vi "Motors.vi"() -> ()   [LabVIEW 2017]
uses:
  <vilib>/Utility/miscctls.llb/LV3DPointTypeDef.ctl
  <vilib>/HaroTek/Haro3D/Utilities/3D objects/controls/Material_info.ctl
  <vilib>/HaroTek/Haro3D/Utilities/3D objects/Box_class/3D_Box.lvclass
  C:/Program Files (x86)/National Instruments/LabVIEW 2017/vi.lib/HaroTek/Haro3D/Utilities/3D objects/3D_Shape_class/3D_Shape.lvclass
  <vilib>/HaroTek/Haro3D/Utilities/3D objects/Cylinder_class/3D_Cylinder.lvclass
  <vilib>/HaroTek/Haro3D/Utilities/3D objects/Sphere_class/3D_Sphere_class/3D_Sphere.lvclass
  <vilib>/HaroTek/Haro3D/Utilities/3D objects/3D_Quad_class/Panel.lvclass
  <vilib>/picture/3D Picture Control/Object/Create Object (name).vi
  <vilib>/picture/3D Picture Control/Object/Add Object (no reference).vi
  <vilib>/HaroTek/Haro3D/Hololens/Hololens_class/Hololens.lvclass
  <vilib>/HaroTek/Haro3D/Hololens/Modules/Hololens Message classes/Text_Message_class/Text_Message.lvclass
  <vilib>/HaroTek/Haro3D/Haro3D.lvlib
  <vilib>/picture/3D Picture Control/NI_3D Picture Control.lvlib
panel:
  in  "TestVar":dbl
  in  "Stop Button":bool
  out "Hololens ON?":bool
  out "3D Picture":refnum<vi>(3d-picture)
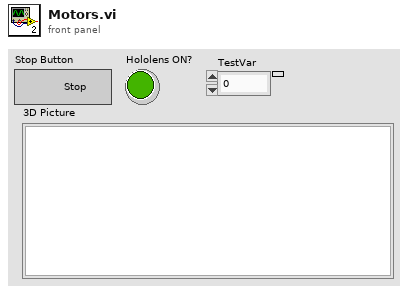
[diagram p1: front panel]
types:
  T1 = typedef "Haro3D.lvlib/Hololens.lvclass/Hololens_event.ctl" = cluster{"Connection":refnum<user-event>, "Data":refnum<user-event>}
  T2 = typedef "LV3DPointTypeDef.ctl" = cluster{"X":sgl, "Y":sgl, "Z":sgl}
  T3 = typedef "Haro3D.lvlib/Material_info.ctl" = cluster{"name":string, "Ka":u32, "Kd":u32, "Ke":u32, "Ks":u32, "map_Ka":string, "map_Kd":string, "map_Ks":string, "Ns":sgl, "Tr":sgl, "UseTexture":bool}
  T4 = typedef "Haro3D.lvlib/Hololens.lvclass/data_event_type.ctl" = enum32{"None", "Mesh", "Text Response", "Manipulation", "Object selected", "Hold", "Receive Anchor", "Sharing", "Secondary connect", "Receive Picture", "Invalid"}
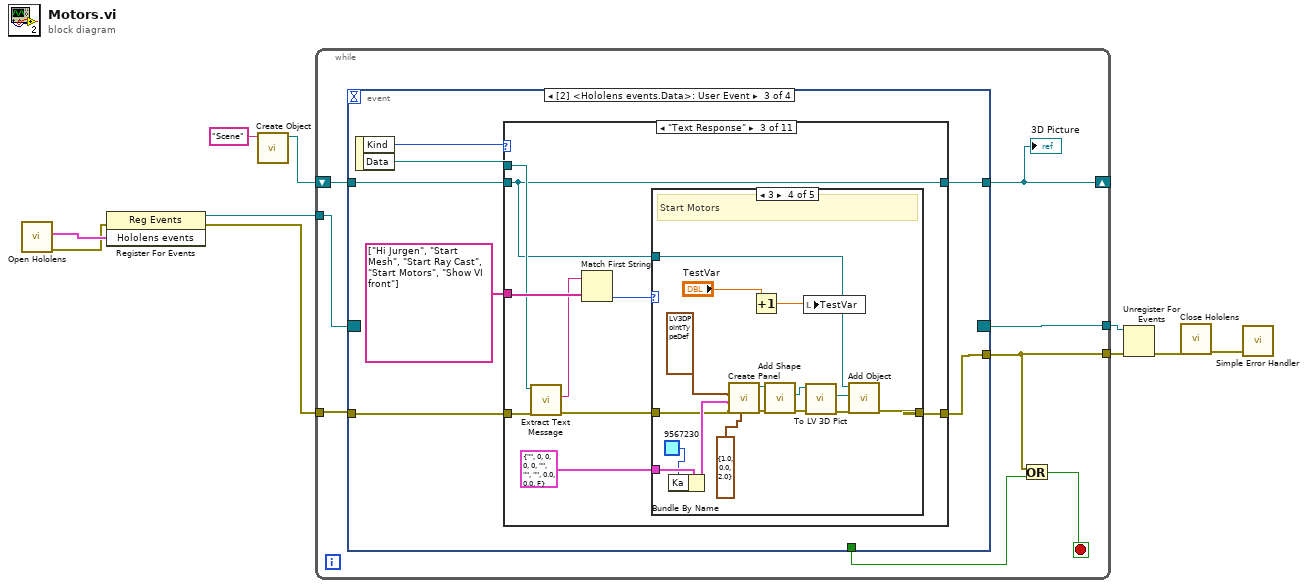
[diagram p0: block diagram]
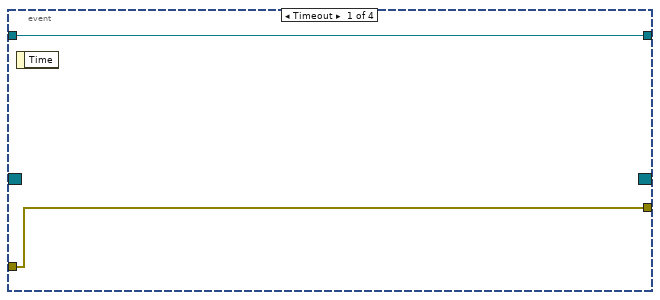
[diagram p2: hidden frame]
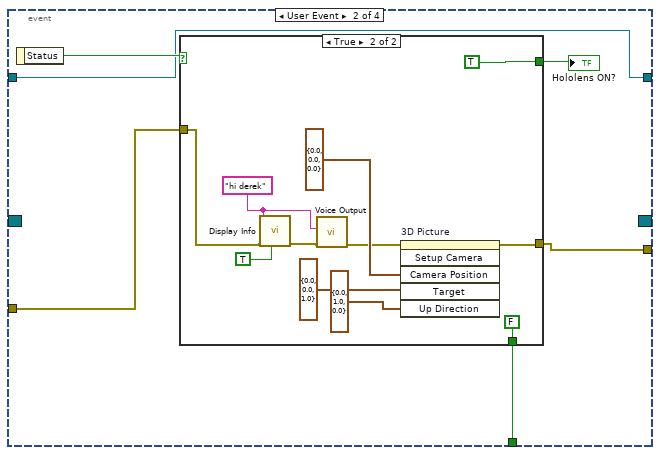
[diagram p3: hidden frame]
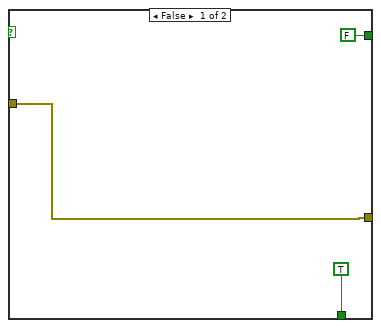
[diagram p4: hidden frame]
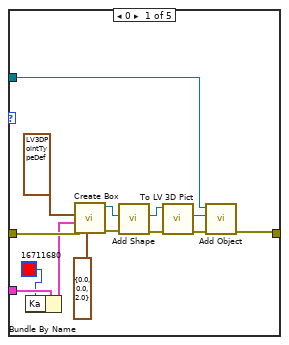
[diagram p7: hidden frame]
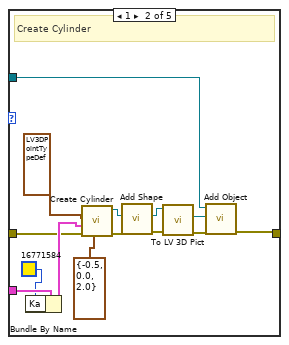
[diagram p8: hidden frame]
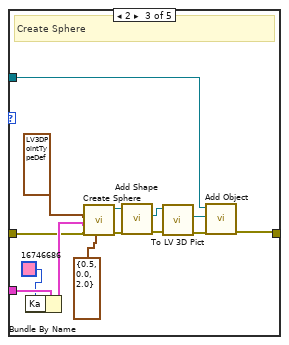
[diagram p9: hidden frame]
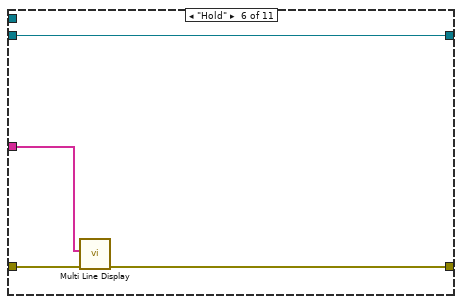
[diagram p13: hidden frame]
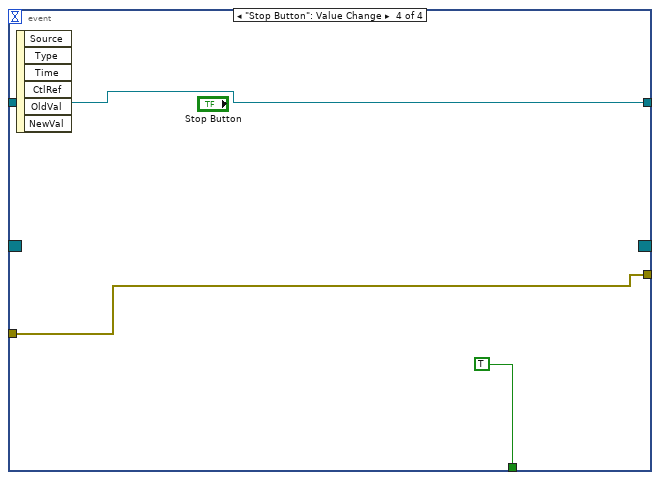
[diagram p19: hidden frame]
diagram:
  n1 = call <vilib>:"Open Hololens.vi"() -> ("error out"=w9:errorcluster, "Hololens events"=w10:T1)  [unwired: 10 in]
  n2 = register-events(error in=w9, w10) -> (reference out=w8:refnum<event-registration>, error out=w7:errorcluster)  [unwired: 1 in]
  n3 = call-poly <vilib>:"Create Object.vi"("Name"="Scene") -> ("Scene:New Object"=w1:refnum<vi>)  [unwired: 9 in, 1 out]
  n4 = while {
    tunnel: w8 -> [w18]
    tunnel: w7 -> [w17]
    tunnel: [w14] -> w6
    tunnel: [w16] -> w4
    shift-right: [w11] -> _
    shift-left: w1 -> [w12]
    stop <- w13 stop-if-true
    n5 = event shown="[2] <Hololens events.Data>: User Event" {
      selector: w18 -> [_ _ _ _]
      dyn-events: [_ _ _ _] -> w16
      timeout: _ -> [_ _ _ _]
      tunnel: w17 -> [w19 w25 w46 w140]
      tunnel: [_ w23 _ TRUE] -> w15
      tunnel: [w19 w22 w44 w140] -> w14
      tunnel: w12 -> [w20 w21 w42 w138]
      tunnel: [w20 w21 w41 w138] -> w11
      event Timeout {
        n6 = event-data() -> ()  [unwired: 1 in, 1 out]
      }
      event User Event {
        n7 = event-data() -> ("Status"=w26:bool)  [unwired: 1 in]
        n8 = case shown="True" w26 {
          tunnel: w25 -> [w28 w37]
          tunnel: [FALSE TRUE] -> w24
          tunnel: [w28 w32] -> w22
          tunnel: [TRUE FALSE] -> w23
          frame False {
          }
          frame True {
            w38 = "hi derek" ("Text to display")
            n9 = call <vilib>:"Display Info.vi"("1 Button?"=TRUE, "error in (no error)"=w37, "Text to display"=w38) -> ("error out"=w39:errorcluster)  [unwired: 8 in]
            n10 = call <vilib>:"Voice Output.vi"("error in (no error)"=w39, "Voice message"=w38) -> ("error out"=w30:errorcluster)  [unwired: 9 in]
            n11 = invoke on="3D Picture" class="SceneGraphDisp (strict)" method="Setup Camera"(error in=w30, "Camera Position"=T2 {"X"=0.0, "Y"=0.0, "Z"=0.0}, "Target"=T2 {"X"=0.0, "Y"=0.0, "Z"=1.0}, "Up Direction"=T2 {"X"=0.0, "Y"=1.0, "Z"=0.0}) -> (error out=w32:errorcluster)  [unwired: 2 in, 5 out]
          }
        }
        "Hololens ON?" <- w24
      }
      event User Event {
        n12 = event-data() -> ("Kind"=w47:T4, "Data"=w43:refnum<class "Holo_Event_Data.lvclass">)  [unwired: 1 in]
        n13 = case shown="\"Text Response\"" w47 {
          tunnel: w46 -> [w48 w50 w59 w120 w122 w127 w128 w130 w132 w134 w136]
          tunnel: string[] ["Hi Jurgen", "Start Mesh", "Start Ray Cast", "Start Motors", "Show VI front"] ("Text lines") -> [_ _ w60 _ _ w126 _ _ _ _ _]
          tunnel: [w48 w50 w55 w120 w122 w125 w128 w130 w132 w134 w136] -> w44
          tunnel: w43 -> [_ _ w58 _ _ _ _ _ _ _ _]
          tunnel: w42 -> [w49 w51 w52 w121 w123 w124 w129 w131 w133 w135 w137]
          tunnel: [w49 w51 w52 w121 w123 w124 w129 w131 w133 w135 w137] -> w41
          frame "None" {
          }
          frame "Mesh" {
          }
          frame "Text Response" {
            n14 = call <vilib>:"Extract Text Message.vi"("error in (no error)"=w59, "Generic Event Message"=w58) -> ("error out"=w54:errorcluster, "Text out"=w57:string)  [unwired: 7 in, 1 out]
            n15 = Match First String(2:w60, 3:w57) -> (0:w56:i32)  [unwired: 1 out]
            n16 = case shown="3" w56 {
              tunnel: [w62 w86 w100 w116 w119] -> w55
              tunnel: w54 -> [w73 w81 w91 w107 w119]
              tunnel: T3 {"name"="", "Ka"=0, "Kd"=0, "Ke"=0, "Ks"=0, "map_Ka"="", "map_Kd"="", "map_Ks"="", "Ns"=0.0, "Tr"=0.0, "UseTexture"=FALSE} ("Material info") -> [w72 w88 w102 w118 _]
              tunnel: w52 -> [w61 w85 w99 w115 _]
              frame 0 {
                n17 = Bundle By Name(cluster=w72, "Ka"=u32 16711680) -> (w71:T3)
                n18 = call <vilib>:"Create Box.vi"("Position"=T2 {"X"=0.0, "Y"=0.0, "Z"=2.0}, "error in (no error)"=w73, "Material info"=w71, "Dimensions"=T2 {"X"=0.3, "Y"=0.2, "Z"=0.1}) -> ("error out"=w68:errorcluster, "Box out"=w67:refnum<class "3D_Box.lvclass">)  [unwired: 6 in]
                n19 = call <vilib>:"Add Shape.vi"("error in (no error)"=w68, "Shape in"=w67) -> ("error out"=w66:errorcluster, "Shape out"=w65:refnum<class "3D_Box.lvclass">)  [unwired: 7 in, 1 out]
                n20 = call-dynamic "To LV 3D Pict.vi"("error in (no error)"=w66, "Box in"=w65) -> ("error out"=w64:errorcluster, "3D object ref"=w63:refnum<vi>)  [unwired: 7 in, 1 out]
                n21 = call-poly <vilib>:"Add Object.vi"("error in (no error)"=w64, "New Object In"=w63, "Scene Object In"=w61) -> ("error out"=w62:errorcluster)  [unwired: 7 in, 1 out]
              }
              frame 1 {
                # "Create Cylinder"
                n22 = Bundle By Name(cluster=w88, "Ka"=u32 16771584) -> (w82:T3)
                n23 = call <vilib>:"Create Cylinder.vi"("Position"=T2 {"X"=-0.5, "Y"=0.0, "Z"=2.0}, "error in (no error)"=w81, "Material info"=w82, "Dimensions"=T2 {"X"=0.3, "Y"=0.1, "Z"=0.1}) -> ("error out"=w84:errorcluster, "Cylinder out"=w75:refnum<class "3D_Cylinder.lvclass">)  [unwired: 6 in]
                n24 = call <vilib>:"Add Shape.vi"("error in (no error)"=w84, "Shape in"=w75) -> ("error out"=w79:errorcluster, "Shape out"=w78:refnum<class "3D_Cylinder.lvclass">)  [unwired: 7 in, 1 out]
                n25 = call-dynamic "To LV 3D Pict.vi"("error in (no error)"=w79, "Cylinder in"=w78) -> ("error out"=w76:errorcluster, "3D object ref"=w77:refnum<vi>)  [unwired: 7 in, 1 out]
                n26 = call-poly <vilib>:"Add Object.vi"("error in (no error)"=w76, "New Object In"=w77, "Scene Object In"=w85) -> ("error out"=w86:errorcluster)  [unwired: 7 in, 1 out]
              }
              frame 2 {
                # "Create Sphere"
                n27 = Bundle By Name(cluster=w102, "Ka"=u32 16746686) -> (w92:T3)
                n28 = call <vilib>:"Create Sphere.vi"("Position"=T2 {"X"=0.5, "Y"=0.0, "Z"=2.0}, "error in (no error)"=w91, "Material info"=w92, "Dimensions"=T2 {"X"=0.3, "Y"=0.3, "Z"=0.3}) -> ("error out"=w94:errorcluster, "Sphere out"=w89:refnum<class "3D_Sphere.lvclass">)  [unwired: 6 in]
                n29 = call <vilib>:"Add Shape.vi"("error in (no error)"=w94, "Shape in"=w89) -> ("error out"=w98:errorcluster, "Shape out"=w97:refnum<class "3D_Sphere.lvclass">)  [unwired: 7 in, 1 out]
                n30 = call-dynamic "To LV 3D Pict.vi"("error in (no error)"=w98, "Sphere in"=w97) -> ("error out"=w95:errorcluster, "LabVIEW 3D object ref"=w96:refnum<vi>)  [unwired: 7 in, 1 out]
                n31 = call-poly <vilib>:"Add Object.vi"("error in (no error)"=w95, "New Object In"=w96, "Scene Object In"=w99) -> ("error out"=w100:errorcluster)  [unwired: 7 in, 1 out]
              }
              frame 3 {
                # "Start Motors"
                n32 = Bundle By Name(cluster=w118, "Ka"=u32 9567230) -> (w108:T3)
                n33 = call <vilib>:"Create Panel.vi"("Position (0,0,0)"=T2 {"X"=1.0, "Y"=0.0, "Z"=2.0} ("Position"), "error in (no error)"=w107, "Material info (gray)"=w108, "Dimensions"=T2 {"X"=0.3, "Y"=0.3, "Z"=0.3}) -> ("error out"=w110:errorcluster, "Panel object"=w105:refnum<class "Panel.lvclass">)  [unwired: 6 in]
                n34 = Increment(x="TestVar") -> (x+1=w104:dbl)
                n35 = call <vilib>:"Add Shape.vi"("error in (no error)"=w110, "Shape in"=w105) -> ("error out"=w114:errorcluster, "Shape out"=w113:refnum<class "Panel.lvclass">)  [unwired: 7 in, 1 out]
                n36 = local write "TestVar"(w104) -> ()
                n37 = call-dynamic "To LV 3D Pict.vi"("error in (no error)"=w114, "reference in"=w113) -> ("error out"=w111:errorcluster, "3D object ref"=w112:refnum<vi>)  [unwired: 7 in, 1 out]
                n38 = call-poly <vilib>:"Add Object.vi"("error in (no error)"=w111, "New Object In"=w112, "Scene Object In"=w115) -> ("error out"=w116:errorcluster)  [unwired: 7 in, 1 out]
              }
              frame Default {
              }
            }
          }
          frame "Manipulation" {
          }
          frame "Object selected" {
          }
          frame "Hold" {
            n39 = call <vilib>:"Multi Line Display.vi"("error in (no error)"=w127, "Text lines"=w126) -> ("error out"=w125:errorcluster)  [unwired: 9 in]
          }
          frame "Receive Anchor" {
          }
          frame "Sharing" {
          }
          frame "Secondary connect" {
          }
          frame "Receive Picture" {
          }
          frame "Invalid" {
          }
        }
      }
      event "Stop Button": Value Change {
        n40 = event-data() -> ()  [unwired: 1 in, 6 out]
      }
    }
    "3D Picture" <- w11
    n41 = Or(x=w14, y=w15) -> (x .or. y?=w13:bool)
  }
  n42 = Unregister For Events(event registration refnum=w4, error in=w6) -> (error out=w5:errorcluster)
  n43 = call <vilib>:"Close Hololens.vi"("error in (no error)"=w5) -> ("error out"=w3:errorcluster)  [unwired: 10 in]
  n44 = call <vilib>:"Simple Error Handler.vi"("error in (no error)"=w3) -> ()  [unwired: 4 in, 5 out]
